vi "未命名 2.vi"(0 "Image In":T1, 1 "Image Dst":T1, 7 "error in":errorcluster) -> (20 "Image Out":T1, 27 "error out":errorcluster)   [LabVIEW 2017]
doc: "Creates, edits, and runs vision algorithms using NI Vision Assistant.\n\nWhen you place this Express VI on the block diagram, NI Vision Assistant launches. Create an algorithm using the Vision Assistant processing functions. After you create an algorithm, you can select the controls and indicators that you want to be able to programmatically set in LabVIEW. Double-click the Vision Assistant Express VI to edit the algorithm."
uses:
  <vilib>/vision/Image Controls.llb/IMAQ Image.ctl
  <vilib>/vision/NI_Vision_Development_Module.lvlib
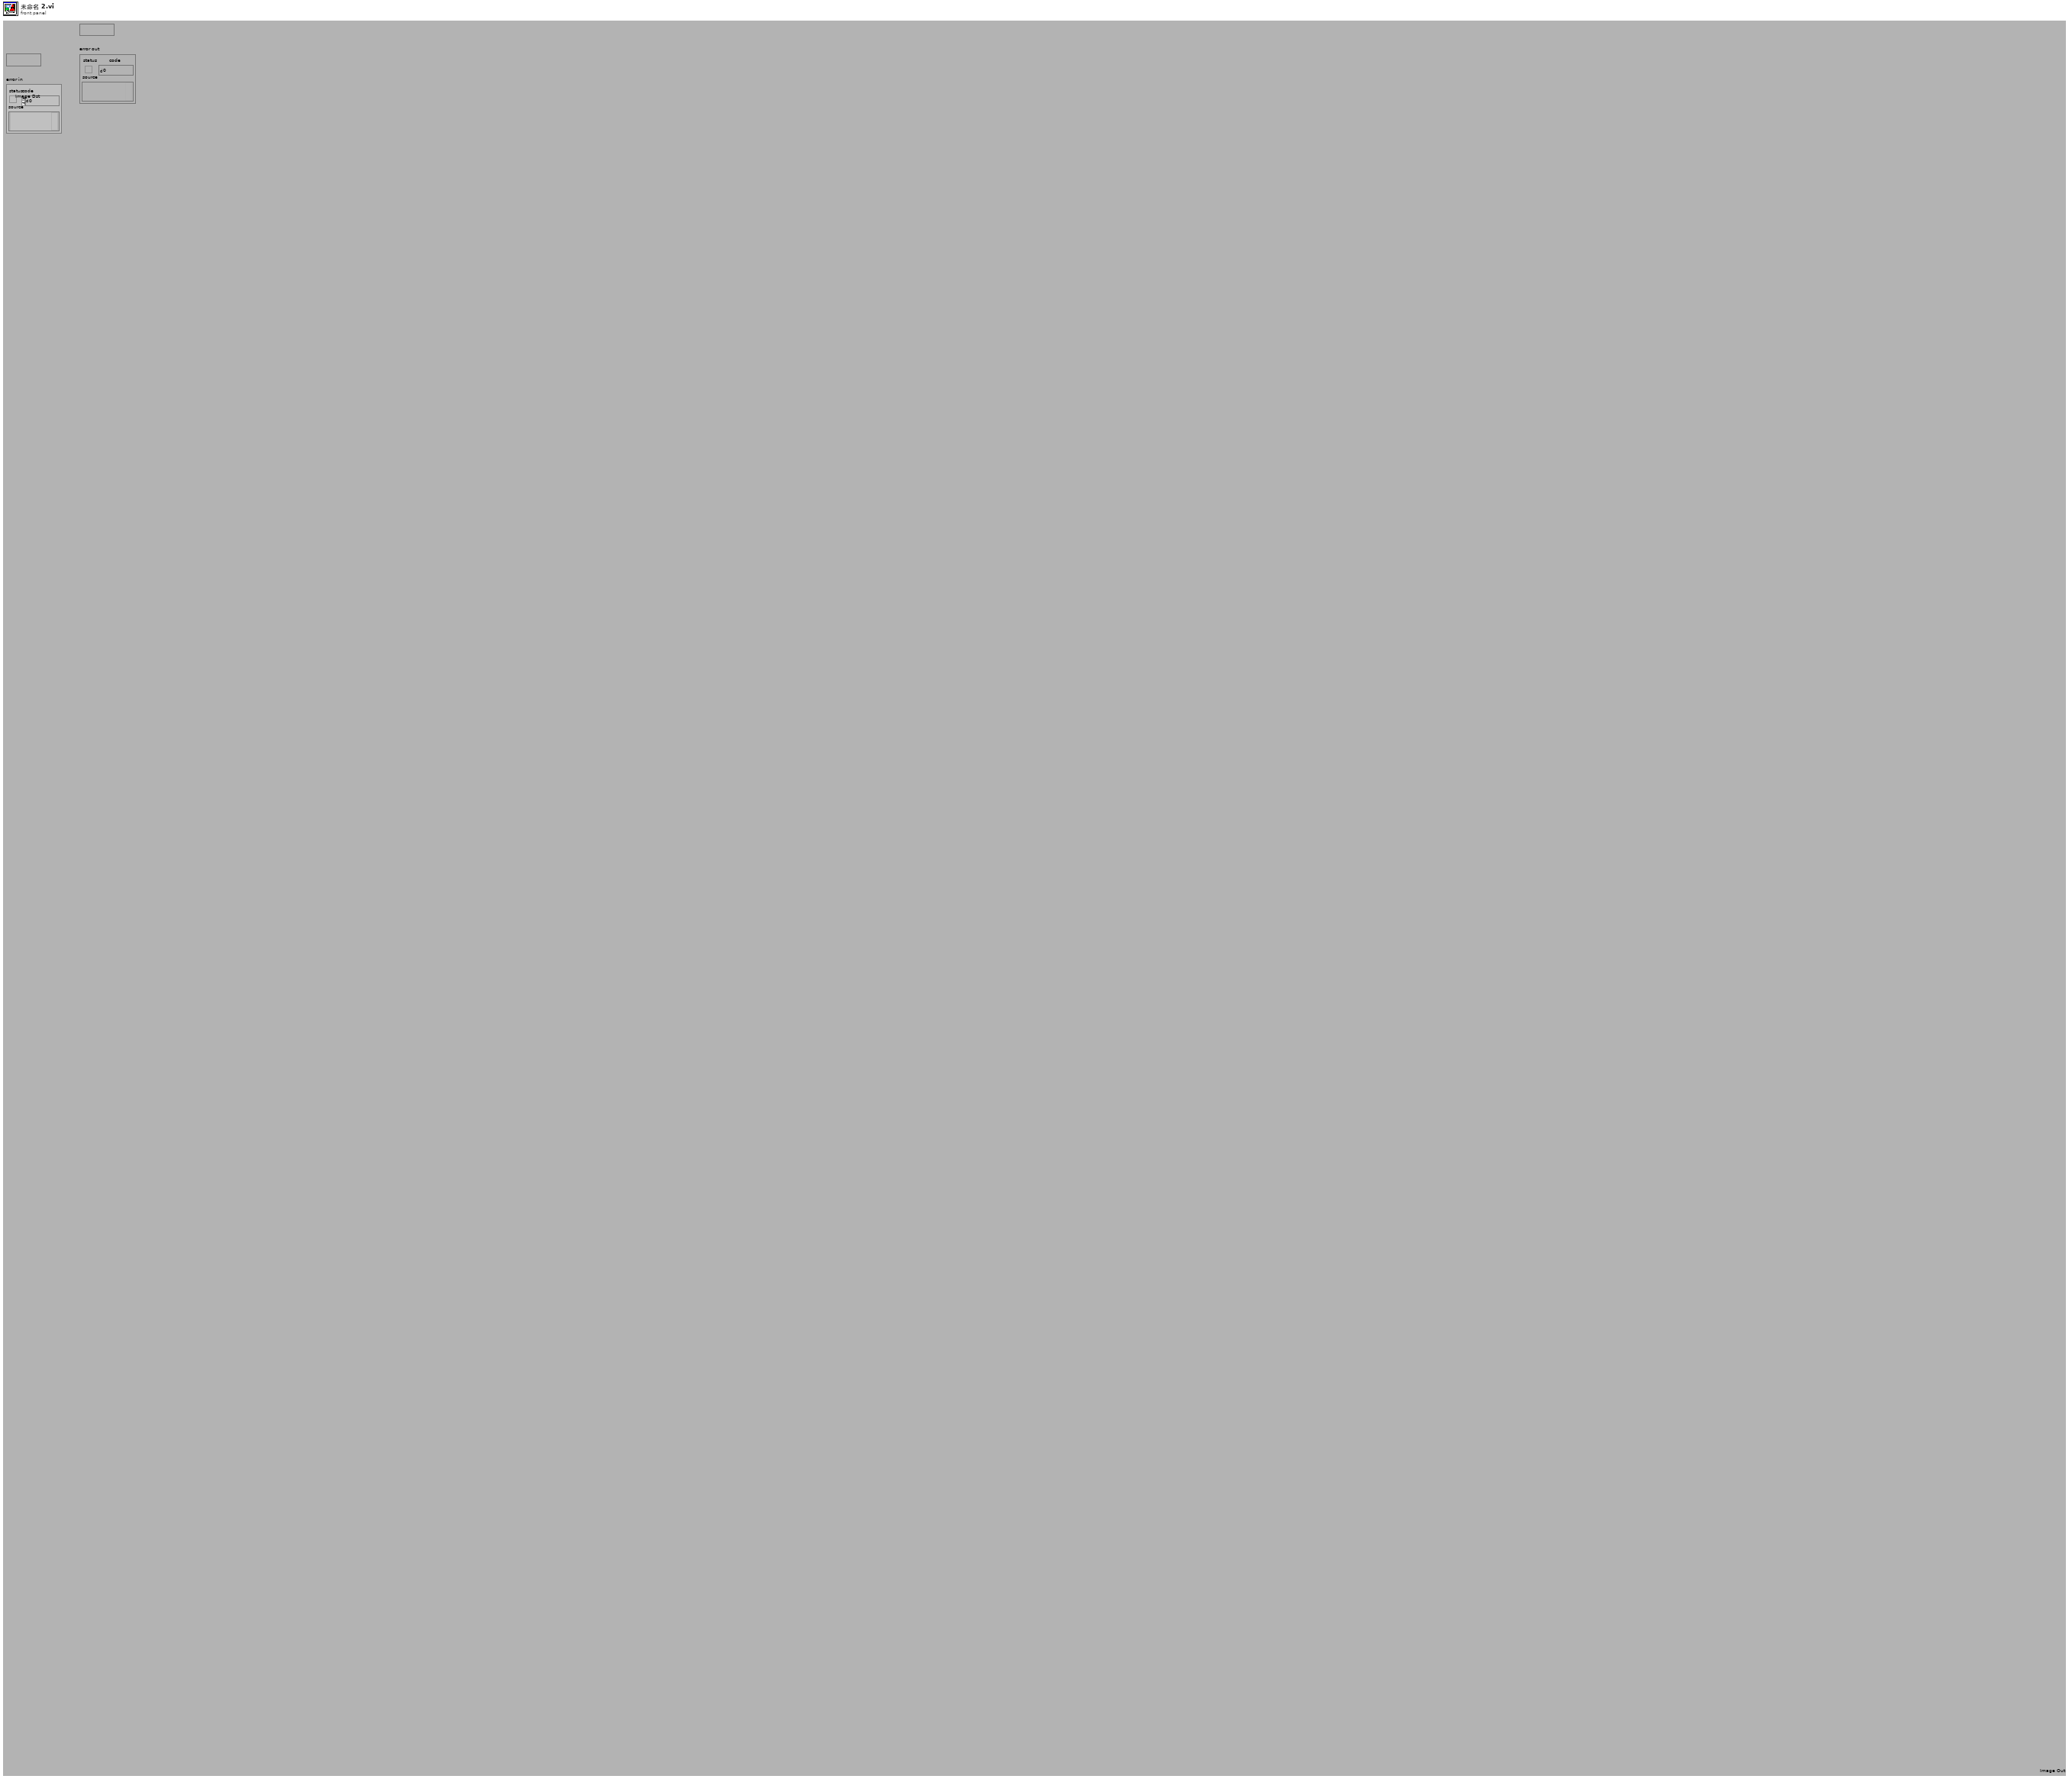
[diagram p1: front panel]
types:
  T1 = typedef "IMAQ Image.ctl" = refnum<image>
  T2 = enum16{"Reset", "Update Coordinate System", "Get Coordinate System"}
  T3 = enum16{"Horizontal Motion", "Vertical Motion", "Horizontal and Vertical Motion", "Horizontal, Vertical and Angular Motion"}
  T4 = cluster{"Origin":cluster{"X":sgl, "Y":sgl}, "Angle (deg)":sgl, "Axis Reference":u32}
  T5 = cluster{"Number of Matches Requested":i32, "Minimum Match Score":sgl, "Angle Ranges":cluster{"Start Angle":sgl, "End Angle":sgl}[]}
  T6 = cluster{"Global Rectangle":i32[], "Contours":cluster{"ID":enum32{"External", "Internal"}, "Type":u32, "Coordinates":i32[]}[]}
  T7 = typedef "Image Type" = u32
  T8 = cluster{"Position":cluster{"x":sgl, "y":sgl}, "Angle":sgl, "Scale":sgl, "Score":sgl, "Bounding Box":cluster{"x":sgl, "y":sgl}[]}[]
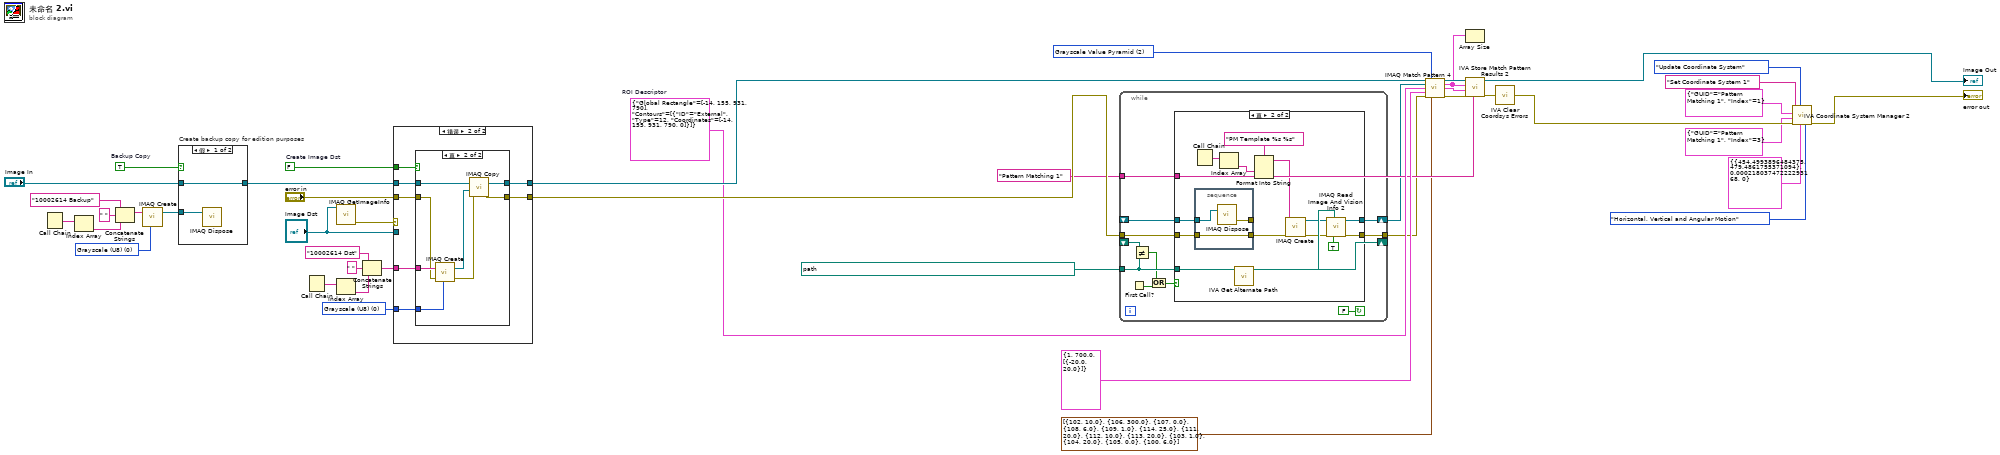
[diagram p0: block diagram]
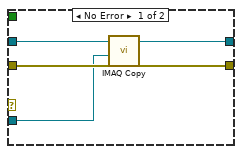
[diagram p3: hidden frame]
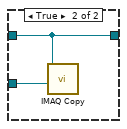
[diagram p5: hidden frame]
diagram:
  w19 = 2 items=["All", "Low Discrepancy Sampling", "Grayscale Value Pyramid", "Gradients Pyramid"] ("Algorithm")
  w16 = "Pattern Matching 1" ("Step Name")
  w18 = T6 {"Global Rectangle"=[-14, 155, 931, 790], "Contours"=[{"ID"=enum."External", "Type"=12, "Coordinates"=[-14, 155, 931, 790, 0]}]}  # ROI Descriptor
  w24 = T7 0 items=["Grayscale (U8)", "Grayscale (I16)", "Grayscale (SGL)", "Complex (CSG)", "RGB (U32)", "HSL (U32)", "RGB (U64)", "Grayscale (U16)"] ("Image Dst Type")
  w25 = T7 0 items=["Grayscale (U8)", "Grayscale (I16)", "Grayscale (SGL)", "Complex (CSG)", "RGB (U32)", "HSL (U32)", "RGB (U64)", "Grayscale (U16)"] ("Image Type")
  w44 = TRUE  # Backup Copy
  w37 = FALSE  # Create Image Dst
  n1 = Call Chain() -> (call chain=w31:string[])
  n2 = Index Array(array=w31) -> (element=w30:string)  [unwired: 1 in]
  n3 = Concatenate Strings("10002614 Backup" ("Backup Image Name"), " ", w30) -> (w27:string)
  n4 = call "IMAQ Create"("Image Name"=w27, "Image Type"=w25) -> ("New Image"=w26:T1)  [unwired: 2 in, 2 out]
  n5 = case "Create backup copy for edition purposes" shown="假" w44 {
    tunnel: [w46 w48] -> w40
    tunnel: "Image In" -> [w46 w48]
    tunnel: w26 -> [w45 w47]
    frame False {
      n6 = call "IMAQ Dispose"("Image"=w45) -> ()  [unwired: 2 in, 4 out]
    }
    frame True {
      n7 = call "IMAQ Copy"("Image Dst"=w47, "Image Src"=w48) -> ()  [unwired: 1 in, 5 out]
    }
  }
  n8 = Call Chain() -> (call chain=w36:string[])
  n9 = call "IMAQ GetImageInfo"("Image"="Image Dst") -> ("error out"=w42:errorcluster)  [unwired: 1 in, 9 out]
  n10 = Index Array(array=w36) -> (element=w34:string)  [unwired: 1 in]
  n11 = Concatenate Strings("10002614 Dst" ("Image Dst Name"), " ", w34) -> (w32:string)
  n12 = case "条件结构" shown="错误" w42 {
    tunnel: [w53 w57] -> w22
    tunnel: [w52 w56] -> w38
    tunnel: w40 -> [w51 w58]
    tunnel: "error in" -> [w50 w54]
    tunnel: "Image Dst" -> [w49 _]
    tunnel: w32 -> [_ w60]
    tunnel: w24 -> [_ w59]
    tunnel: w37 -> [_ w55]
    frame No Error {
      n13 = call "IMAQ Copy"("error in (no error)"=w50, "Image Dst"=w49, "Image Src"=w51) -> ("error out"=w52:errorcluster, "Image Dst Out"=w53:T1)  [unwired: 3 out]
    }
    frame Error {
      n14 = case "条件结构" shown="真" w55 {
        tunnel: w60 -> [_ w70]
        tunnel: w59 -> [_ w69]
        tunnel: w58 -> [w62 w67]
        tunnel: [w62 w66] -> w57
        tunnel: [w61 w65] -> w56
        tunnel: w54 -> [w61 w63]
        frame False {
        }
        frame True {
          n15 = call "IMAQ Create"("Image Name"=w70, "Image Type"=w69, "error in (no error)"=w63) -> ("New Image"=w68:T1, "error out"=w64:errorcluster)  [unwired: 1 in, 1 out]
          n16 = call "IMAQ Copy"("error in (no error)"=w64, "Image Dst"=w68, "Image Src"=w67) -> ("error out"=w65:errorcluster, "Image Dst Out"=w66:T1)  [unwired: 3 out]
        }
      }
    }
  }
  n17 = while {
    shift-right: [w81] -> w13
    shift-left: _ -> [w80]
    tunnel: [w78] -> w12
    tunnel: w38 -> [w77]
    tunnel: path "D:/Inspect System/Source Code/Template Program/字符检测定位模板.png" ("Template File Path") -> [w74]
    tunnel: w16 -> [w76]
    shift-right: [w74] -> _
    shift-left: _ -> [w75]
    stop <- FALSE continue-if-true
    n18 = First Call?() -> (First Call?: T/F=w73:bool)
    n19 = Not Equal?(x=w75, y=w74) -> (x != y?=w72:bool)
    n20 = Or(x=w72, y=w73) -> (x .or. y?=w71:bool)
    n21 = case "条件结构" shown="真" w71 {
      tunnel: [w83 w88] -> w81
      tunnel: w80 -> [w83 w92]
      tunnel: [w82 w89] -> w78
      tunnel: w77 -> [w82 w91]
      tunnel: w74 -> [_ w93]
      tunnel: w76 -> [_ w94]
      frame False {
      }
      frame True {
        n22 = stacked-sequence "层叠式顺序结构" {
          tunnel: w92 -> [w101]
          tunnel: w91 -> [w100]
          tunnel: [w100] -> w85
          tunnel: [w99] -> _
          frame #0 {
            n23 = call "IMAQ Dispose"("Image"=w101) -> ("error out"=w99:errorcluster)  [unwired: 2 in, 3 out]
          }
        }
        n24 = Call Chain() -> (call chain=w96:string[])
        n25 = Index Array(array=w96) -> (element=w95:string)  [unwired: 1 in]
        n26 = call <vilib>:"IVA Get Alternate Path.vi"("Path In"=w93) -> ("Path Out"=w90:path)  [unwired: 10 out]
        n27 = Format Into String(format string="PM Template %s %s" ("Image Name"), w95, w94) -> (resulting string=w98:string)  [unwired: 2 in, 1 out]
        n28 = call "IMAQ Create"("Image Name"=w98, "error in (no error)"=w85) -> ("New Image"=w87:T1, "error out"=w86:errorcluster)  [unwired: 2 in, 1 out]
        n29 = call "IMAQ Read Image And Vision Info 2"("Use File Path Image Type"=TRUE, "File Path"=w90, "error in (no error)"=w86, "Image"=w87) -> ("error out"=w89:errorcluster, "Image Out"=w88:T1)  [unwired: 5 in, 1 out]
      }
    }
  }
  n30 = call "IMAQ Match Pattern 4"("Image"=w22, "Algorithm"=w19, "Template Image"=w13, "ROI Descriptor"=w18, "Parameters"=T5 {"Number of Matches Requested"=1, "Minimum Match Score"=700.0, "Angle Ranges"=[{"Start Angle"=-20.0, "End Angle"=20.0}]}, "error in (no error)"=w12, "Advanced Options"=cluster{"Item":u16, "Value":dbl}[] [{"Item"=102, "Value"=10.0}, {"Item"=106, "Value"=300.0}, {"Item"=107, "Value"=0.0}, {"Item"=108, "Value"=6.0}, {"Item"=109, "Value"=1.0}, {"Item"=114, "Value"=25.0}, {"Item"=111, "Value"=20.0}, {"Item"=112, "Value"=10.0}, {"Item"=113, "Value"=20.0}, {"Item"=103, "Value"=1.0}, {"Item"=104, "Value"=20.0}, {"Item"=105, "Value"=0.0}, {"Item"=100, "Value"=6.0}]) -> ("Image (duplicate)"=w20:T1, "Matches (pixel)"=w15:T8, "Matches (real-world)"=w14:T8, "error out"=w21:errorcluster)  [unwired: 4 in, 1 out]
  n31 = Array Size(array=w15) -> ()  [unwired: 1 out]
  n32 = call <vilib>:"IVA Store Match Pattern Results 2.vi"("Step Name"=w16, "error in (no error)"=w21, "Matches (real-world)"=w14, "Matches (pixel)"=w15, "Image in"=w20) -> ("error out"=w11:errorcluster, "Image dup"=→"Image Out":T1)  [unwired: 1 in, 4 out]
  n33 = call <vilib>:"IVA Clear Coordsys Errors.vi"("error in (no error)"=w11) -> ("error out"=w10:errorcluster)  [unwired: 10 in]
  n34 = call <vilib>:"IVA Coordinate System Manager 2.vi"("Mode"=T3."Horizontal, Vertical and Angular Motion", "Reference System"=T4 {"Origin"={"X"=454.4994, "Y"=479.48618}, "Angle (deg)"=0.00021803747, "Axis Reference"=0}, "Function"=T2."Update Coordinate System", "error in (no error)"=w10, "Angle ID"=cluster{"GUID":string, "Index":i32} {"GUID"="Pattern Matching 1", "Index"=3}, "Origin ID"=cluster{"GUID":string, "Index":i32} {"GUID"="Pattern Matching 1", "Index"=1}, "Coordinate System Name"="Set Coordinate System 1") -> ("error out"=→"error out":errorcluster)  [unwired: 4 out]
